vi "Query Integrate Status.vi"(8 "error in (no error)":errorcluster, 10 "Element (1)":i32(ring)=1 items=["1"=1, "2"=2, "3"=3, "4"=4, "5"=5, "6"=6], 11 "VISA resource name":refnum<visa-resource-name>) -> (0 "error out":errorcluster, 1 "Integrate Status List":bool[](array[boolean]), 2 "Integrate Status":i32, 3 "VISA resource name out":refnum<visa-resource-name>)   [LabVIEW 2021, in "Yokogawa WT1800 Series.lvlib"]
doc: "Queries the integration status."
uses:
  <instrlib>/Yokogawa WT1800 Series/Yokogawa WT1800 Series.lvlib
panel:
  # "Reset"
  # "Ready"
  # "Start"
  # "Stop"
  # "Error"
  # "Time up"
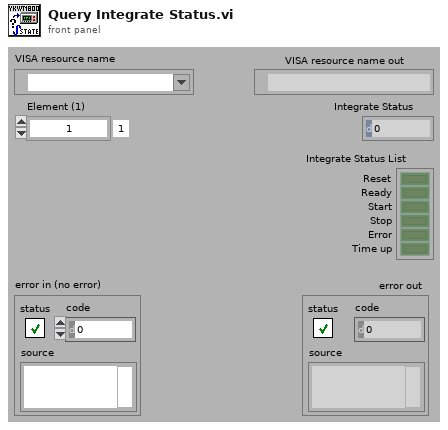
[diagram p1: front panel]
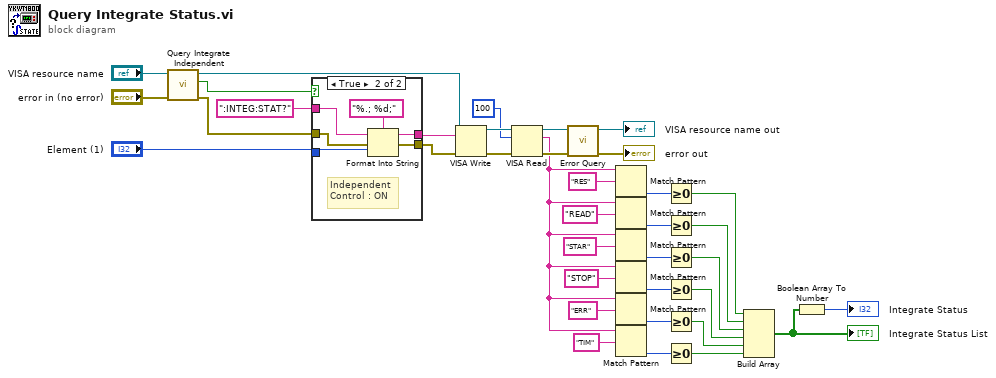
[diagram p0: block diagram]
diagram:
  n1 = call <instrlib>:"Query Integrate Independent.vi"("error in (no error)"="error in (no error)", "VISA resource name"="VISA resource name") -> ("error out"=w2:errorcluster, "Independent Control"=w1:bool, "VISA resource name out"=w4:refnum<visa-resource-name>)  [unwired: 7 in]
  n2 = case shown="True" w1 {
    tunnel: "Element (1)" -> [_ w44]
    tunnel: [w39 w43] -> w31
    tunnel: w2 -> [w38 w42]
    tunnel: [w38 w41] -> w30
    tunnel: ":INTEG:STAT?" ("形式文字列") -> [w39 w40]
    frame False {
      # "Independent\nControl : OFF"
    }
    frame True {
      # "Independent\nControl : ON"
      n3 = Format Into String(format string="%.; %d;" ("形式文字列"), initial string=w40, error in=w42, w44) -> (resulting string=w43:string, error out=w41:errorcluster)
    }
  }
  n4 = VISA Write ("VISA書き込み")(VISA resource name=w4, write buffer=w31, error in (no error)=w30) -> (VISA resource name out=w36:refnum<visa-resource-name>, error out=w37:errorcluster)  [unwired: 1 out]
  n5 = VISA Read ("VISA読み取り")(VISA resource name=w36, byte count=u32 100, error in (no error)=w37) -> (VISA resource name out=w34:refnum<visa-resource-name>, read buffer=w22:string, error out=w28:errorcluster)  [unwired: 1 out]
  n6 = call <instrlib>:"Error Query.vi"("error in (no error)"=w28, "VISA resource name"=w34) -> ("error out"=→"error out":errorcluster, "VISA resource name out"=→"VISA resource name out":refnum<visa-resource-name>)  [unwired: 6 in, 2 out]
  n7 = Match Pattern(string=w22, regular expression="RES") -> (offset past match=w21:i32)  [unwired: 1 in, 3 out]
  n8 = Match Pattern(string=w22, regular expression="READ") -> (offset past match=w19:i32)  [unwired: 1 in, 3 out]
  n9 = Match Pattern(string=w22, regular expression="STAR") -> (offset past match=w18:i32)  [unwired: 1 in, 3 out]
  n10 = Match Pattern(string=w22, regular expression="STOP") -> (offset past match=w17:i32)  [unwired: 1 in, 3 out]
  n11 = Match Pattern(string=w22, regular expression="ERR") -> (offset past match=w16:i32)  [unwired: 1 in, 3 out]
  n12 = Match Pattern(string=w22, regular expression="TIM") -> (offset past match=w20:i32)  [unwired: 1 in, 3 out]
  n13 = Greater Or Equal To 0?(x=w21) -> (x >= 0?=w10:bool)
  n14 = Greater Or Equal To 0?(x=w19) -> (x >= 0?=w11:bool)
  n15 = Greater Or Equal To 0?(x=w18) -> (x >= 0?=w12:bool)
  n16 = Greater Or Equal To 0?(x=w17) -> (x >= 0?=w13:bool)
  n17 = Greater Or Equal To 0?(x=w16) -> (x >= 0?=w14:bool)
  n18 = Greater Or Equal To 0?(x=w20) -> (x >= 0?=w15:bool)
  n19 = Build Array(w10, w11, w12, w13, w14, w15) -> (w9:bool[])
  "Integrate Status List" <- w9
  n20 = Boolean Array To Number(Boolean array=w9) -> (number=→"Integrate Status":u32)
